vi "写入map.vi"(8 "error in (no error)":errorcluster caption="错误输入（无错误）", 10 "map":u8[][](array[numeric]), 11 "生命游戏输入":refnum<class "生命游戏.lvclass">) -> (0 "error out":errorcluster caption="错误输出", 3 "生命游戏输出":refnum<class "生命游戏.lvclass">)   [LabVIEW 2015, in "生命游戏.lvlib" / "生命游戏.lvclass"]
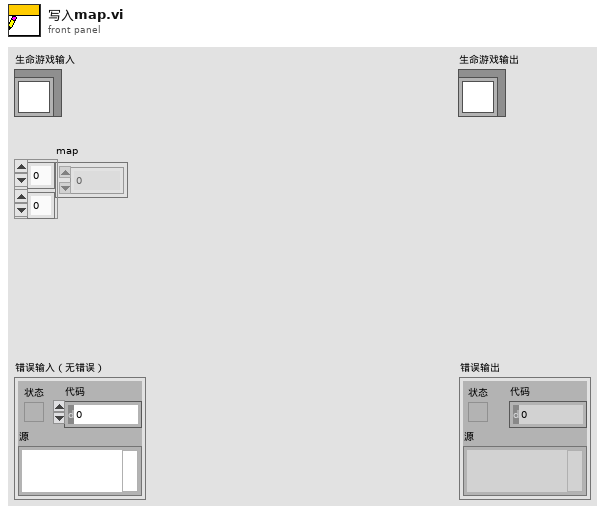
[diagram p1: front panel]
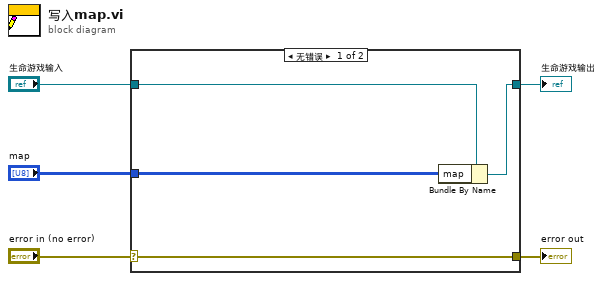
[diagram p0: block diagram]
diagram:
  n1 = case shown="无错误" "error in (no error)" {
    selector: "error in (no error)" -> [w9 w10]
    tunnel: [w9 w10] -> w4
    tunnel: [w7 w11] -> w2
    tunnel: "生命游戏输入" -> [w8 w11]
    tunnel: "map" -> [w6 _]
    frame No Error {
      n2 = Bundle By Name(cluster=w8, "map"=w6) -> (w7:refnum<class "生命游戏.lvclass">)
    }
    frame Error {
    }
  }
  "error out" <- w4
  "生命游戏输出" <- w2
